vi "EOL CAN_Update CAL.vi"(8 "Glass?":bool=TRUE, 9 "Read Session in":refnum<k21>, 10 "DSC Write Session in":refnum<k21>, 11 "Download Parameter":T1) -> (1 "Error String Out":string, 2 "TxRx Data":string[][](array[string]), 3 "Response Good?":bool)   [LabVIEW 2014]
uses:
  Typedefs/Select Session.ctl
  <vilib>/xnet/xnet.llb/XNET Frame CAN.ctl
  <vilib>/xnet/xnet.llb/XNET Frame Type CAN.ctl
  <vilib>/xnet/xnet.llb/XNET Read (Frame CAN).vi
panel:
  in  "Error String":string
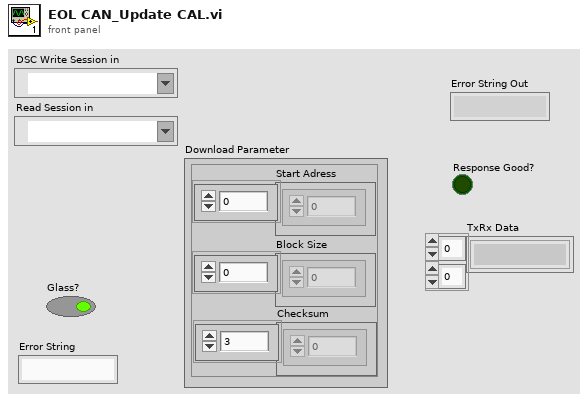
[diagram p1: front panel]
types:
  T1 = cluster{"Start Adress":u8[], "Block Size":u8[], "Checksum":u8[]}
  T2 = cluster{"DSC Write Session in":refnum<k21>, "Read Session in":refnum<k21>, "Error String":string, "Response Good?":bool, "Glass?":bool, "TxRx Data":string[][], "Download Parameter":cluster{"Start Adress":u8[], "Block Size":u8[], "Checksum":u8[]}}
  T3 = typedef "Select Session.ctl" = enum16{"DefaultSession", "Development", "Extended", "EOL", "Programming"}
  T4 = typedef "XNET Frame CAN.ctl" = cluster{"timestamp":timestamp, "payload":u8[], "identifier":u32, "type":T5, "extended?":bool, "echo?":bool}
  T5 = typedef "XNET Frame Type CAN.ctl" = u8
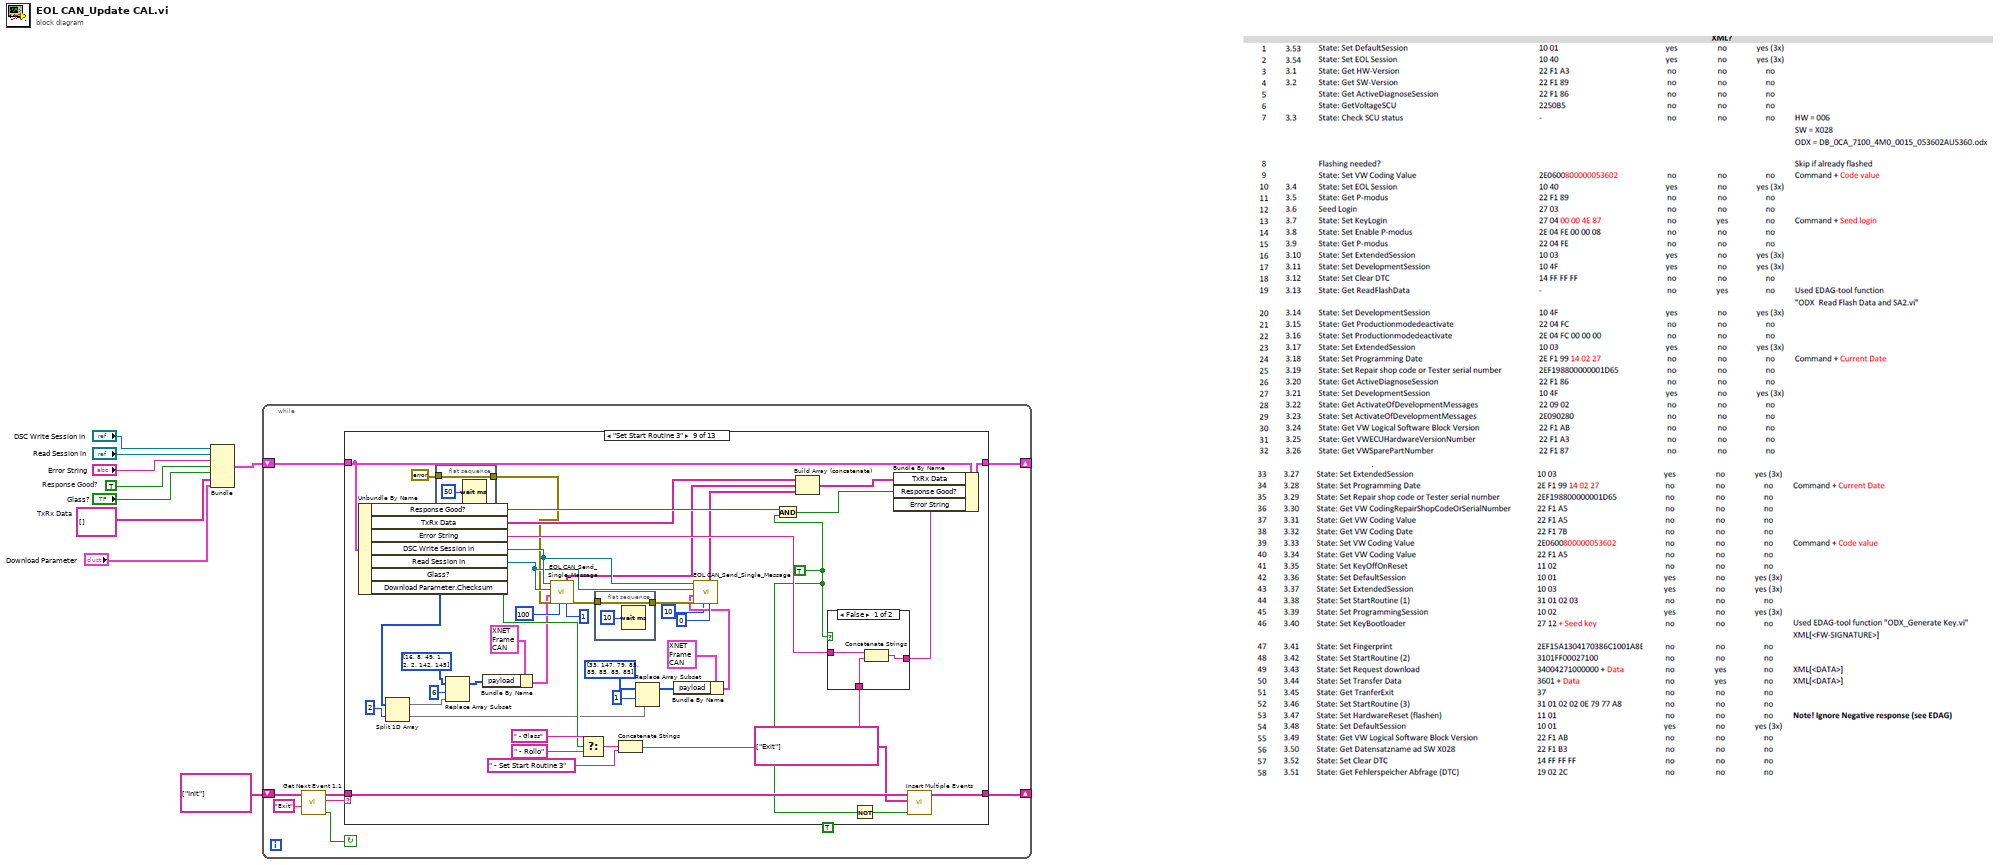
[diagram p0: block diagram]
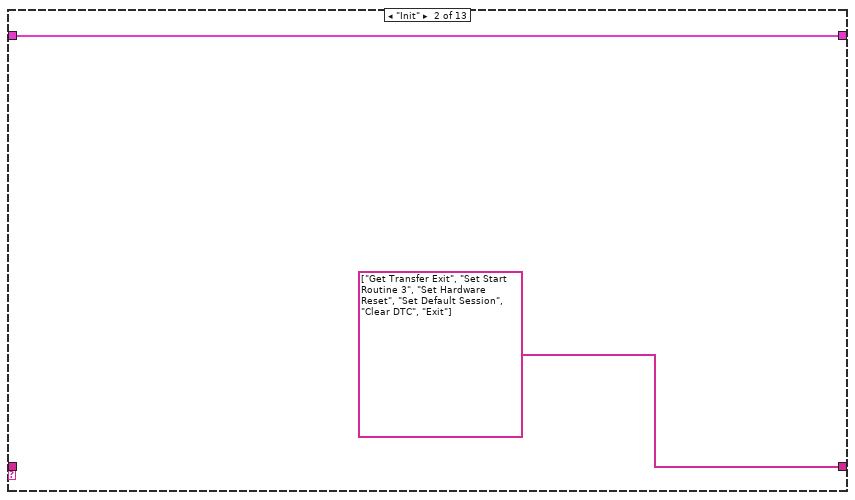
[diagram p3: hidden frame]
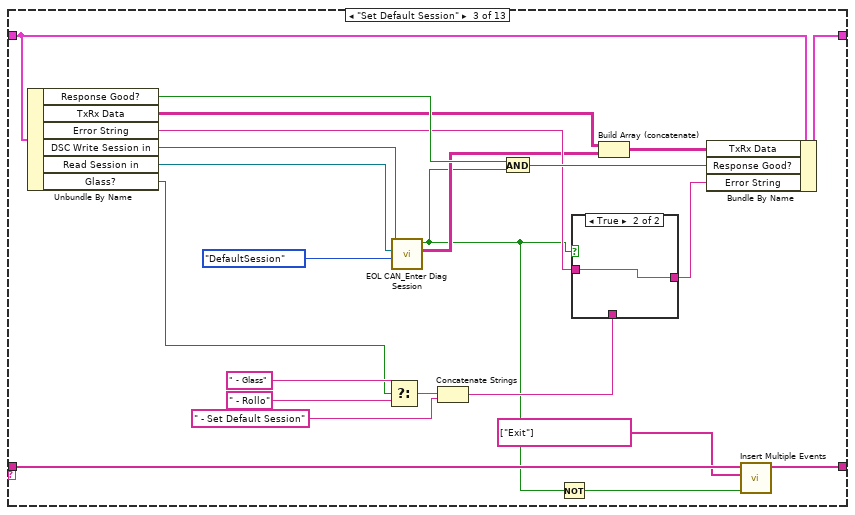
[diagram p4: hidden frame]
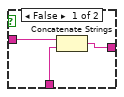
[diagram p5: hidden frame]
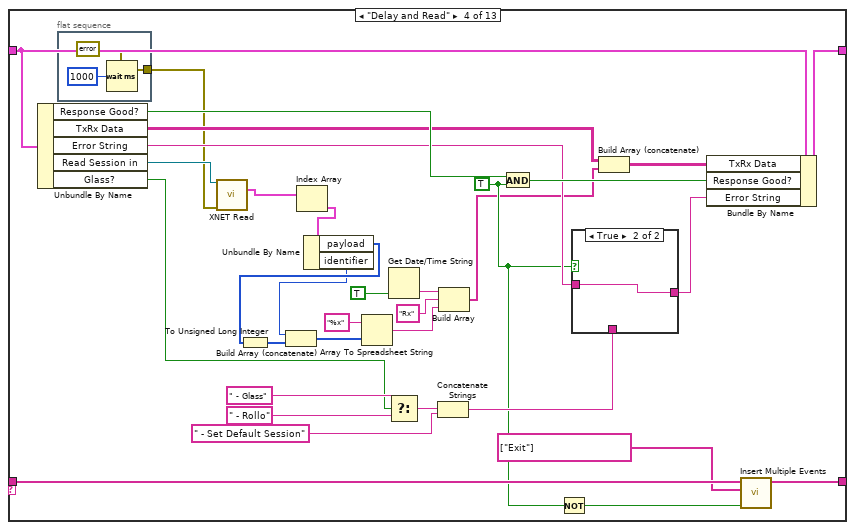
[diagram p6: hidden frame]
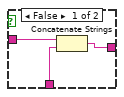
[diagram p7: hidden frame]
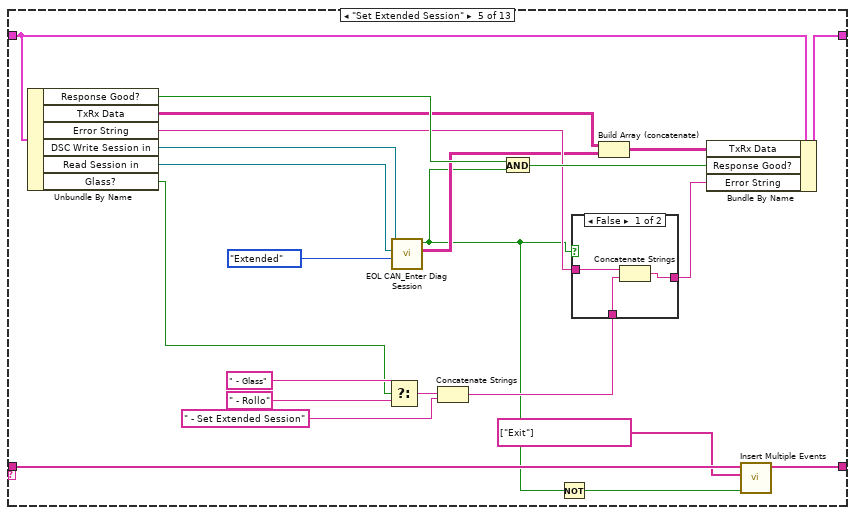
[diagram p8: hidden frame]
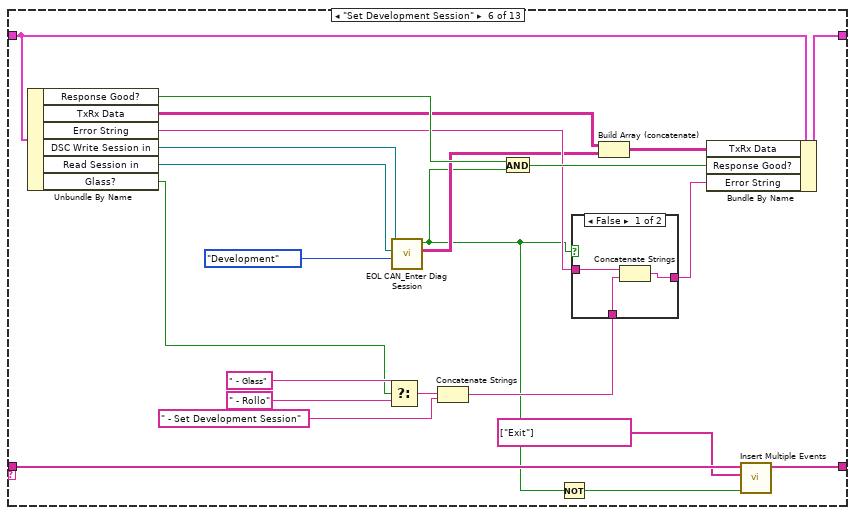
[diagram p10: hidden frame]
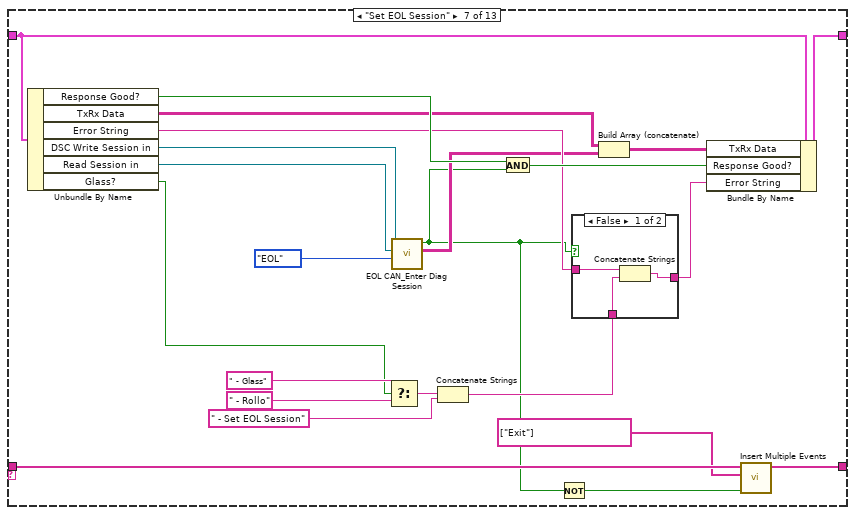
[diagram p12: hidden frame]
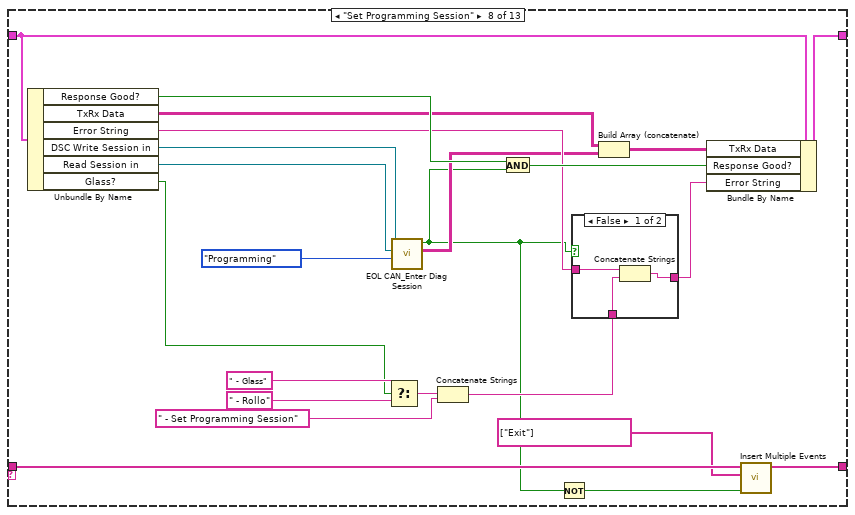
[diagram p14: hidden frame]
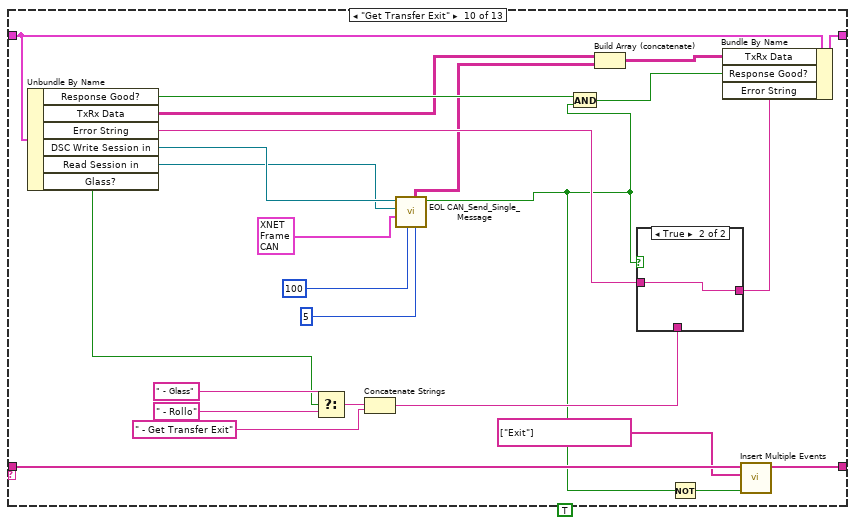
[diagram p17: hidden frame]
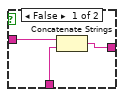
[diagram p18: hidden frame]
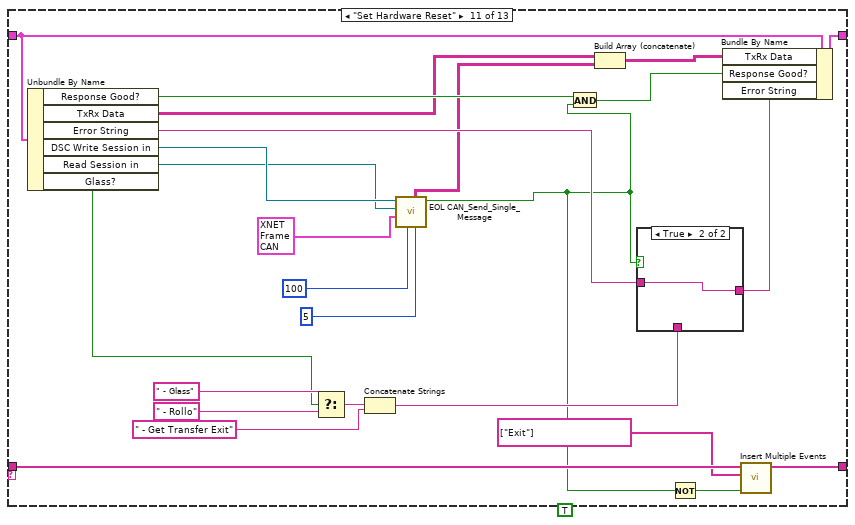
[diagram p19: hidden frame]
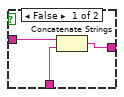
[diagram p20: hidden frame]
diagram:
  w4 = string[][] []  # TxRx Data
  w7 = TRUE  # Response Good?
  n1 = Bundle("DSC Write Session in"="DSC Write Session in", "Read Session in"="Read Session in", "Error String"="Error String", "Response Good?"=w7, "Glass?"="Glass?", "TxRx Data"=w4, "Download Parameter"="Download Parameter") -> (w6:T2)  [unwired: 1 in]
  n2 = while {
    shift-right: [w15] -> _
    shift-left: string[] ["Init"] ("event queue out") -> [w14]
    shift-right: [w12] -> _
    shift-left: w6 -> [w13]
    stop <- w17 continue-if-true
    n3 = call "Get Next Event 1.1.vi"("Exit Event"="Exit", "event queue in"=w14) -> ("Condition (Exit:F)"=w17:bool, "next event"=w10:string, "event queue out"=w16:string[])  [unwired: 6 in, 1 out]
    n4 = case shown="\"Set Start Routine 3\"" w10 {
      tunnel: w16 -> [w19 _ w32 w69 w98 w125 w152 w179 w228 w261 w290 w316 w337]
      tunnel: [w19 string[] ["Get Transfer Exit", "Set Start Routine 3", "Set Hardware Reset", "Set Default Session", "Clear DTC", "Exit"] ("event queue out") w33 w70 w99 w126 w153 w180 w229 w262 w291 w317 w337] -> w15
      tunnel: w13 -> [w18 w21 w43 w80 w109 w136 w163 w190 w239 w272 w301 w327 w336]
      tunnel: [w18 w21 w41 w78 w107 w134 w161 w188 w237 w270 w299 w325 w336] -> w12
      frame "Error", Default {
      }
      frame "Init" {
      }
      frame "Set Default Session" {
        n5 = Unbundle By Name(w43) -> ("Response Good?"=w44:bool, "TxRx Data"=w30:string[][], "Error String"=w40:string, "DSC Write Session in"=w27:refnum<k21>, "Read Session in"=w26:refnum<k21>, "Glass?"=w24:bool)
        n6 = Select(t=" - Glass" ("Error Description"), s=w24, f=" - Rollo" ("Error Description")) -> (s? t:f=w38:string)
        n7 = call "EOL CAN_Enter Diag Session.vi"("Session"=Select_Session."DefaultSession", "Read Session in"=w26, "Write Session in"=w27) -> ("TxRx Data"=w28:string[][], "Response Good?"=w23:bool)  [unwired: 6 in, 1 out]
        n8 = Concatenate Strings(w38, " - Set Default Session" ("Error Description")) -> (w34:string)
        n9 = And(x=w44, y=w23) -> (x .and. y?=w42:bool)
        n10 = Not(x=w23) -> (.not. x?=w22:bool)
        n11 = case shown="True" w23 {
          tunnel: w40 -> [w46 w48]
          tunnel: [w47 w48] -> w39
          tunnel: w34 -> [w45 _]
          frame False {
            n12 = Concatenate Strings(w46, w45) -> (w47:string)
          }
          frame True {
          }
        }
        n13 = Build Array (concatenate)(w30, w28) -> (w29:string[][])
        n14 = Bundle By Name(cluster=w43, "TxRx Data"=w29, "Response Good?"=w42, "Error String"=w39) -> (w41:T2)
        n15 = call "Insert Multiple Events.vi"("Insert all? (T)"=w22, "Events to Insert"=string[] ["Exit"], "Event queue in"=w32) -> ("Event queue out"=w33:string[])  [unwired: 4 in]
      }
      frame "Delay and Read" {
        w62 = TRUE ("y")
        n16 = Unbundle By Name(w80) -> ("Response Good?"=w81:bool, "TxRx Data"=w67:string[][], "Error String"=w77:string, "Read Session in"=w63:refnum<k21>, "Glass?"=w65:bool)
        n17 = flat-sequence {
          tunnel: [errorcluster {"status"=FALSE, "code"=0, "source"=""} ("error out")] -> w49
          frame #0 {
            n18 = Wait (ms)(milliseconds to wait=u32 1000) -> ()  [unwired: 1 out]
          }
        }
        n19 = call-poly <vilib>:"XNET Read.vi"("session in"=w63, "error in (no error)"=w49) -> ("data"=w53:T4[])  [unwired: 10 in, 3 out]
        n20 = Index Array(array=w53) -> (element=w52:T4)  [unwired: 1 in]
        n21 = Unbundle By Name(w52) -> ("payload"=w51:u8[], "identifier"=w50:u32)
        n22 = To Unsigned Long Integer(number=w51) -> (unsigned 32bit integer=w61:u32[])
        n23 = Build Array (concatenate)(w50, w61) -> (w55:u32[])
        n24 = Array To Spreadsheet String(array=w55, 3:"%x" ("format string")) -> (spreadsheet string=w56:string)  [unwired: 1 in]
        n25 = Get Date/Time String(want seconds? (F)=TRUE) -> (time string=w58:string)  [unwired: 2 in, 1 out]
        n26 = Select(t=" - Glass" ("Error Description"), s=w65, f=" - Rollo" ("Error Description")) -> (s? t:f=w75:string)
        n27 = Concatenate Strings(w75, " - Set Default Session" ("Error Description")) -> (w71:string)
        n28 = Build Array(w58, "Rx" ("format string"), w56) -> (w54:string[])
        n29 = And(x=w81, y=w62) -> (x .and. y?=w79:bool)
        n30 = Not(x=w62) -> (.not. x?=w64:bool)
        n31 = case shown="True" w62 {
          tunnel: w77 -> [w85 w87]
          tunnel: [w86 w87] -> w76
          tunnel: w71 -> [w84 _]
          frame False {
            n32 = Concatenate Strings(w85, w84) -> (w86:string)
          }
          frame True {
          }
        }
        n33 = Build Array (concatenate)(w67, w54) -> (w66:string[][])
        n34 = Bundle By Name(cluster=w80, "TxRx Data"=w66, "Response Good?"=w79, "Error String"=w76) -> (w78:T2)
        n35 = call "Insert Multiple Events.vi"("Insert all? (T)"=w64, "Events to Insert"=string[] ["Exit"], "Event queue in"=w69) -> ("Event queue out"=w70:string[])  [unwired: 4 in]
      }
      frame "Set Extended Session" {
        n36 = Unbundle By Name(w109) -> ("Response Good?"=w110:bool, "TxRx Data"=w96:string[][], "Error String"=w106:string, "DSC Write Session in"=w93:refnum<k21>, "Read Session in"=w92:refnum<k21>, "Glass?"=w90:bool)
        n37 = Select(t=" - Glass" ("Error Description"), s=w90, f=" - Rollo" ("Error Description")) -> (s? t:f=w104:string)
        n38 = call "EOL CAN_Enter Diag Session.vi"("Session"=Select_Session."Extended", "Read Session in"=w92, "Write Session in"=w93) -> ("TxRx Data"=w94:string[][], "Response Good?"=w89:bool)  [unwired: 6 in, 1 out]
        n39 = Concatenate Strings(w104, " - Set Extended Session" ("Error Description")) -> (w100:string)
        n40 = And(x=w110, y=w89) -> (x .and. y?=w108:bool)
        n41 = Not(x=w89) -> (.not. x?=w88:bool)
        n42 = case shown="False" w89 {
          tunnel: w106 -> [w112 w114]
          tunnel: [w113 w114] -> w105
          tunnel: w100 -> [w111 _]
          frame False {
            n43 = Concatenate Strings(w112, w111) -> (w113:string)
          }
          frame True {
          }
        }
        n44 = Build Array (concatenate)(w96, w94) -> (w95:string[][])
        n45 = Bundle By Name(cluster=w109, "TxRx Data"=w95, "Response Good?"=w108, "Error String"=w105) -> (w107:T2)
        n46 = call "Insert Multiple Events.vi"("Insert all? (T)"=w88, "Events to Insert"=string[] ["Exit"], "Event queue in"=w98) -> ("Event queue out"=w99:string[])  [unwired: 4 in]
      }
      frame "Set Development Session" {
        n47 = Unbundle By Name(w136) -> ("Response Good?"=w137:bool, "TxRx Data"=w123:string[][], "Error String"=w133:string, "DSC Write Session in"=w120:refnum<k21>, "Read Session in"=w119:refnum<k21>, "Glass?"=w117:bool)
        n48 = Select(t=" - Glass" ("Error Description"), s=w117, f=" - Rollo" ("Error Description")) -> (s? t:f=w131:string)
        n49 = call "EOL CAN_Enter Diag Session.vi"("Session"=Select_Session."Development", "Read Session in"=w119, "Write Session in"=w120) -> ("TxRx Data"=w121:string[][], "Response Good?"=w116:bool)  [unwired: 6 in, 1 out]
        n50 = Concatenate Strings(w131, " - Set Development Session" ("Error Description")) -> (w127:string)
        n51 = And(x=w137, y=w116) -> (x .and. y?=w135:bool)
        n52 = Not(x=w116) -> (.not. x?=w115:bool)
        n53 = case shown="False" w116 {
          tunnel: w133 -> [w139 w141]
          tunnel: [w140 w141] -> w132
          tunnel: w127 -> [w138 _]
          frame False {
            n54 = Concatenate Strings(w139, w138) -> (w140:string)
          }
          frame True {
          }
        }
        n55 = Build Array (concatenate)(w123, w121) -> (w122:string[][])
        n56 = Bundle By Name(cluster=w136, "TxRx Data"=w122, "Response Good?"=w135, "Error String"=w132) -> (w134:T2)
        n57 = call "Insert Multiple Events.vi"("Insert all? (T)"=w115, "Events to Insert"=string[] ["Exit"], "Event queue in"=w125) -> ("Event queue out"=w126:string[])  [unwired: 4 in]
      }
      frame "Set EOL Session" {
        n58 = Unbundle By Name(w163) -> ("Response Good?"=w164:bool, "TxRx Data"=w150:string[][], "Error String"=w160:string, "DSC Write Session in"=w147:refnum<k21>, "Read Session in"=w146:refnum<k21>, "Glass?"=w144:bool)
        n59 = Select(t=" - Glass" ("Error Description"), s=w144, f=" - Rollo" ("Error Description")) -> (s? t:f=w158:string)
        n60 = call "EOL CAN_Enter Diag Session.vi"("Session"=Select_Session."EOL", "Read Session in"=w146, "Write Session in"=w147) -> ("TxRx Data"=w148:string[][], "Response Good?"=w143:bool)  [unwired: 6 in, 1 out]
        n61 = Concatenate Strings(w158, " - Set EOL Session" ("Error Description")) -> (w154:string)
        n62 = And(x=w164, y=w143) -> (x .and. y?=w162:bool)
        n63 = Not(x=w143) -> (.not. x?=w142:bool)
        n64 = case shown="False" w143 {
          tunnel: w160 -> [w166 w168]
          tunnel: [w167 w168] -> w159
          tunnel: w154 -> [w165 _]
          frame False {
            n65 = Concatenate Strings(w166, w165) -> (w167:string)
          }
          frame True {
          }
        }
        n66 = Build Array (concatenate)(w150, w148) -> (w149:string[][])
        n67 = Bundle By Name(cluster=w163, "TxRx Data"=w149, "Response Good?"=w162, "Error String"=w159) -> (w161:T2)
        n68 = call "Insert Multiple Events.vi"("Insert all? (T)"=w142, "Events to Insert"=string[] ["Exit"], "Event queue in"=w152) -> ("Event queue out"=w153:string[])  [unwired: 4 in]
      }
      frame "Set Programming Session" {
        n69 = Unbundle By Name(w190) -> ("Response Good?"=w191:bool, "TxRx Data"=w177:string[][], "Error String"=w187:string, "DSC Write Session in"=w174:refnum<k21>, "Read Session in"=w173:refnum<k21>, "Glass?"=w171:bool)
        n70 = Select(t=" - Glass" ("Error Description"), s=w171, f=" - Rollo" ("Error Description")) -> (s? t:f=w185:string)
        n71 = call "EOL CAN_Enter Diag Session.vi"("Session"=Select_Session."Programming", "Read Session in"=w173, "Write Session in"=w174) -> ("TxRx Data"=w175:string[][], "Response Good?"=w170:bool)  [unwired: 6 in, 1 out]
        n72 = Concatenate Strings(w185, " - Set Programming Session" ("Error Description")) -> (w181:string)
        n73 = And(x=w191, y=w170) -> (x .and. y?=w189:bool)
        n74 = Not(x=w170) -> (.not. x?=w169:bool)
        n75 = case shown="False" w170 {
          tunnel: w187 -> [w193 w195]
          tunnel: [w194 w195] -> w186
          tunnel: w181 -> [w192 _]
          frame False {
            n76 = Concatenate Strings(w193, w192) -> (w194:string)
          }
          frame True {
          }
        }
        n77 = Build Array (concatenate)(w177, w175) -> (w176:string[][])
        n78 = Bundle By Name(cluster=w190, "TxRx Data"=w176, "Response Good?"=w189, "Error String"=w186) -> (w188:T2)
        n79 = call "Insert Multiple Events.vi"("Insert all? (T)"=w169, "Events to Insert"=string[] ["Exit"], "Event queue in"=w179) -> ("Event queue out"=w180:string[])  [unwired: 4 in]
      }
      frame "Set Start Routine 3" {
        w196 = TRUE
        (unwired) TRUE ("Insert all? (T)")
        n80 = Unbundle By Name(w239) -> ("Response Good?"=w240:bool, "TxRx Data"=w226:string[][], "Error String"=w236:string, "DSC Write Session in"=w223:refnum<k21>, "Read Session in"=w222:refnum<k21>, "Glass?"=w224:bool, "Download Parameter.Checksum"=w201:u8[])
        n81 = Split 1D Array(array=w201, index=2) -> (first subarray=w206:u8[], second subarray=w211:u8[])
        n82 = flat-sequence {
          tunnel: errorcluster {"status"=FALSE, "code"=0, "source"=""} ("Error out") -> [w242]
          tunnel: [w242] -> w214
          frame #0 {
            n83 = Wait (ms)(milliseconds to wait=u32 50) -> ()  [unwired: 1 out]
          }
        }
        n84 = Replace Array Subset(array=u8[] [16, 8, 49, 1, 2, 2, 142, 145] ("payload"), new element=w206, index=6) -> (w204:u8[])
        n85 = Bundle By Name(cluster=T4 {"timestamp"=timestamp(0 s since 1904-01-01), "payload"=[16, 8, 49, 1, 2, 2, 142, 145], "identifier"=402391172, "type"=8, "extended?"=TRUE, "echo?"=FALSE} ("Tx CAN frame"), "payload"=w204) -> (w198:T4)
        n86 = call "EOL CAN_Send_Single_Message.vi"("Retries"=1, "Msg Wait Time"=u32 100, "Error in"=w214, "Tx CAN frame"=w198, "Read Session in"=w222, "Write Session in"=w223) -> ("Error out"=w217:errorcluster, "TxRx Data"=w219:string[][])  [unwired: 1 in, 3 out]
        n87 = Select(t=" - Glass" ("Error Description"), s=w224, f=" - Rollo" ("Error Description")) -> (s? t:f=w234:string)
        n88 = flat-sequence {
          tunnel: w217 -> [w244]
          tunnel: [w244] -> w216
          frame #0 {
            n89 = Wait (ms)(milliseconds to wait=u32 10) -> ()  [unwired: 1 out]
          }
        }
        n90 = Concatenate Strings(w234, " - Set Start Routine 3" ("Error Description")) -> (w230:string)
        n91 = Replace Array Subset(array=u8[] [33, 147, 79, 85, 85, 85, 85, 85] ("payload"), new element=w211, index=1) -> (w208:u8[])
        n92 = Bundle By Name(cluster=T4 {"timestamp"=timestamp(0 s since 1904-01-01), "payload"=[33, 147, 79, 85, 85, 85, 85, 85], "identifier"=402391172, "type"=8, "extended?"=TRUE, "echo?"=FALSE} ("Tx CAN frame"), "payload"=w208) -> (w199:T4)
        n93 = call "EOL CAN_Send_Single_Message.vi"("Retries"=0, "Msg Wait Time"=u32 10, "Error in"=w216, "Tx CAN frame"=w199, "Read Session in"=w222, "Write Session in"=w223) -> ("TxRx Data"=w218:string[][])  [unwired: 1 in, 4 out]
        n94 = And(x=w240, y=w196) -> (x .and. y?=w238:bool)
        n95 = Build Array (concatenate)(w226, w219, w218) -> (w225:string[][])
        n96 = case shown="False" w196 {
          tunnel: w236 -> [w246 w248]
          tunnel: [w247 w248] -> w235
          tunnel: w230 -> [w245 _]
          frame False {
            n97 = Concatenate Strings(w246, w245) -> (w247:string)
          }
          frame True {
          }
        }
        n98 = Not(x=w196) -> (.not. x?=w215:bool)
        n99 = Bundle By Name(cluster=w239, "TxRx Data"=w225, "Response Good?"=w238, "Error String"=w235) -> (w237:T2)
        n100 = call "Insert Multiple Events.vi"("Insert all? (T)"=w215, "Events to Insert"=string[] ["Exit"], "Event queue in"=w228) -> ("Event queue out"=w229:string[])  [unwired: 4 in]
      }
      frame "Get Transfer Exit" {
        (unwired) TRUE ("Insert all? (T)")
        n101 = Unbundle By Name(w272) -> ("Response Good?"=w273:bool, "TxRx Data"=w259:string[][], "Error String"=w269:string, "DSC Write Session in"=w256:refnum<k21>, "Read Session in"=w255:refnum<k21>, "Glass?"=w257:bool)
        n102 = Select(t=" - Glass" ("Error Description"), s=w257, f=" - Rollo" ("Error Description")) -> (s? t:f=w267:string)
        n103 = Concatenate Strings(w267, " - Get Transfer Exit" ("Error Description")) -> (w263:string)
        n104 = call "EOL CAN_Send_Single_Message.vi"("Retries"=5, "Msg Wait Time"=u32 100, "Tx CAN frame"=T4 {"timestamp"=timestamp(0 s since 1904-01-01), "payload"=[1, 55, 85, 85, 85, 85, 85, 85], "identifier"=402391172, "type"=8, "extended?"=TRUE, "echo?"=FALSE}, "Read Session in"=w255, "Write Session in"=w256) -> ("Response Good?"=w249:bool, "TxRx Data"=w252:string[][])  [unwired: 2 in, 3 out]
        n105 = And(x=w273, y=w249) -> (x .and. y?=w271:bool)
        n106 = Build Array (concatenate)(w259, w252) -> (w258:string[][])
        n107 = case shown="True" w249 {
          tunnel: w269 -> [w275 w277]
          tunnel: [w276 w277] -> w268
          tunnel: w263 -> [w274 _]
          frame False {
            n108 = Concatenate Strings(w275, w274) -> (w276:string)
          }
          frame True {
          }
        }
        n109 = Not(x=w249) -> (.not. x?=w250:bool)
        n110 = Bundle By Name(cluster=w272, "TxRx Data"=w258, "Response Good?"=w271, "Error String"=w268) -> (w270:T2)
        n111 = call "Insert Multiple Events.vi"("Insert all? (T)"=w250, "Events to Insert"=string[] ["Exit"], "Event queue in"=w261) -> ("Event queue out"=w262:string[])  [unwired: 4 in]
      }
      frame "Set Hardware Reset" {
        (unwired) TRUE ("Insert all? (T)")
        n112 = Unbundle By Name(w301) -> ("Response Good?"=w302:bool, "TxRx Data"=w288:string[][], "Error String"=w298:string, "DSC Write Session in"=w285:refnum<k21>, "Read Session in"=w284:refnum<k21>, "Glass?"=w286:bool)
        n113 = Select(t=" - Glass" ("Error Description"), s=w286, f=" - Rollo" ("Error Description")) -> (s? t:f=w296:string)
        n114 = Concatenate Strings(w296, " - Get Transfer Exit" ("Error Description")) -> (w292:string)
        n115 = call "EOL CAN_Send_Single_Message.vi"("Retries"=5, "Msg Wait Time"=u32 100, "Tx CAN frame"=T4 {"timestamp"=timestamp(0 s since 1904-01-01), "payload"=[2, 17, 1, 85, 85, 85, 85, 85], "identifier"=402391172, "type"=8, "extended?"=TRUE, "echo?"=FALSE}, "Read Session in"=w284, "Write Session in"=w285) -> ("Response Good?"=w278:bool, "TxRx Data"=w281:string[][])  [unwired: 2 in, 3 out]
        n116 = And(x=w302, y=w278) -> (x .and. y?=w300:bool)
        n117 = Build Array (concatenate)(w288, w281) -> (w287:string[][])
        n118 = case shown="True" w278 {
          tunnel: w298 -> [w304 w306]
          tunnel: [w305 w306] -> w297
          tunnel: w292 -> [w303 _]
          frame False {
            n119 = Concatenate Strings(w304, w303) -> (w305:string)
          }
          frame True {
          }
        }
        n120 = Not(x=w278) -> (.not. x?=w279:bool)
        n121 = Bundle By Name(cluster=w301, "TxRx Data"=w287, "Response Good?"=w300, "Error String"=w297) -> (w299:T2)
        n122 = call "Insert Multiple Events.vi"("Insert all? (T)"=w279, "Events to Insert"=string[] ["Exit"], "Event queue in"=w290) -> ("Event queue out"=w291:string[])  [unwired: 4 in]
      }
      frame "Clear DTC" {
        n123 = Unbundle By Name(w327) -> ("Response Good?"=w328:bool, "TxRx Data"=w314:string[][], "Error String"=w324:string, "DSC Write Session in"=w310:refnum<k21>, "Read Session in"=w309:refnum<k21>, "Glass?"=w312:bool)
        n124 = Select(t=" - Glass" ("Error Description"), s=w312, f=" - Rollo" ("Error Description")) -> (s? t:f=w322:string)
        n125 = Concatenate Strings(w322, " - Clear DTC" ("Error Description")) -> (w318:string)
        n126 = call "EOL CAN_Clear_DTC's.vi"("Read Session in"=w309, "Write Session in"=w310) -> ("TxRx Data"=w308:string[][], "Response Good?"=w307:bool)  [unwired: 7 in, 1 out]
        n127 = And(x=w328, y=w307) -> (x .and. y?=w326:bool)
        n128 = Build Array (concatenate)(w314, w308) -> (w313:string[][])
        n129 = Not(x=w307) -> (.not. x?=w311:bool)
        n130 = case shown="True" w307 {
          tunnel: w324 -> [w330 w332]
          tunnel: [w331 w332] -> w323
          tunnel: w318 -> [w329 _]
          frame False {
            n131 = Concatenate Strings(w330, w329) -> (w331:string)
          }
          frame True {
          }
        }
        n132 = Bundle By Name(cluster=w327, "TxRx Data"=w313, "Response Good?"=w326, "Error String"=w323) -> (w325:T2)
        n133 = call "Insert Multiple Events.vi"("Insert all? (T)"=w311, "Events to Insert"=string[] ["Exit"], "Event queue in"=w316) -> ("Event queue out"=w317:string[])  [unwired: 4 in]
      }
      frame "Exit" {
        n134 = Unbundle By Name(w336) -> ("Response Good?"=→"Response Good?":bool, "Error String"=→"Error String Out":string, "TxRx Data"=→"TxRx Data":string[][])
      }
    }
  }
